vi "Set Local Chassis Apply Module Mode.vi"(8 "error in":errorcluster, 10 "Apply Module Mode":bool, 11 "chassis ref in":T1 format="%.0x") -> (0 "error out":errorcluster, 3 "chassis ref out":T1 format="%.0x")   [LabVIEW 2020, in "Scan Engine Scripting.lvlib"]
doc: "Returns the local chassis name from the provided chassis reference."
uses:
  Scan Engine Scripting.lvlib
  <vilib>/NI VeriStand/Custom Device API/Custom Device Item Ref.ctl
  Shared/Globals/Property Strings.vi
  Shared/SEECD Shared.lvlib
  <vilib>/NI VeriStand/Custom Device API/Custom Device API.lvlib
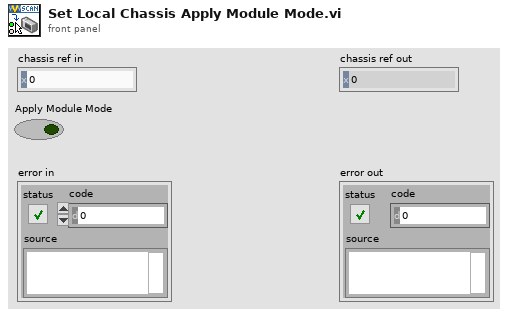
[diagram p1: front panel]
types:
  T1 = typedef "Custom Device API.lvlib/Custom Device Item Ref.ctl" = u64
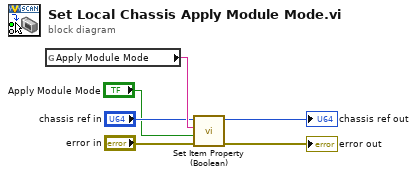
[diagram p0: block diagram]
diagram:
  n1 = global read "Property Strings.vi" "Apply Module Mode"() -> (w4:string)
  n2 = call <vilib>:"Set Item Property (Boolean).vi"("error in (no error)"="error in", "Value"="Apply Module Mode", "Property Name"=w4, "Item Ref in"="chassis ref in") -> ("error out"=→"error out":errorcluster, "Item Ref out"=→"chassis ref out":T1)  [unwired: 5 in, 1 out]
